vi "(Incomplete) Gamma Function.vi"   [LabVIEW 2020, in "NI_Gmath.lvlib"]
doc: "Evaluates the gamma function and regularized incomplete gamma function. You must manually select the polymorphic instance you want to use."
uses:
  NI_Gmath.lvlib
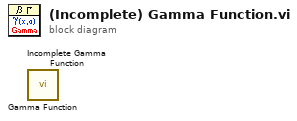
[diagram p0: block diagram]
diagram:
  n1 = call "Gamma Function.vi"() -> ()  [unwired: 11 in, 1 out]
  n2 = call "Incomplete Gamma Function.vi"() -> ()  [unwired: 11 in, 1 out]
